vi "StartSweepMeasurement.vi"(8 "error in (no error)":errorcluster, 11 "9770 API in":refnum<class "9770 API.lvclass">) -> (0 "error out":errorcluster, 3 "9770 API out":refnum<class "9770 API.lvclass">)   [LabVIEW 2017, in "9770 API.lvclass"]
uses:
  <vilib>/addons/InsightCM/Devices/Shared/Emsa/Emsa9770API/9770 API.lvclass
  <vilib>/addons/InsightCM/Devices/Shared/Emsa/Emsa9770API/9770 API.lvclass/9770 API.ctl
  <vilib>/LabVIEW Targets/FPGA/cRIO/shared/nicrio_ModuleControls/nicrio_cRIO-9770_DataRatesRing.ctl
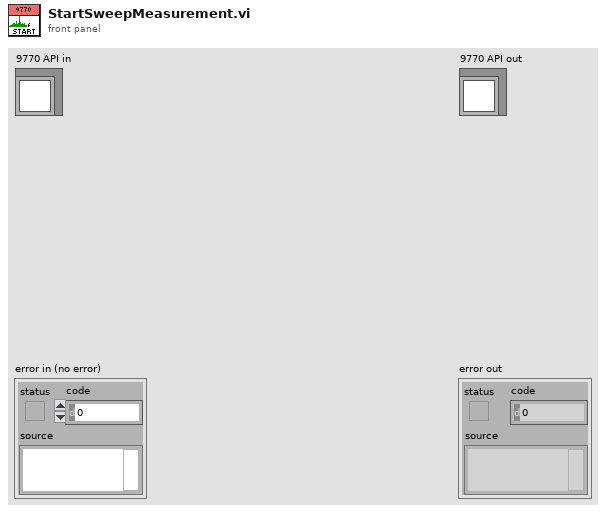
[diagram p1: front panel]
types:
  T1 = cluster{"Sweep":cluster{"Center Freq":dbl, "Bandwidth":dbl}[], "SampleRate":dbl, "FullScaleVoltage":dbl, "DetectionTime":dbl, "DetectionMode":enum16{"Peak", "Quasi Peak", "Average"}}
  T2 = typedef "nicrio_cRIO-9770_DataRatesRing.ctl" = u8
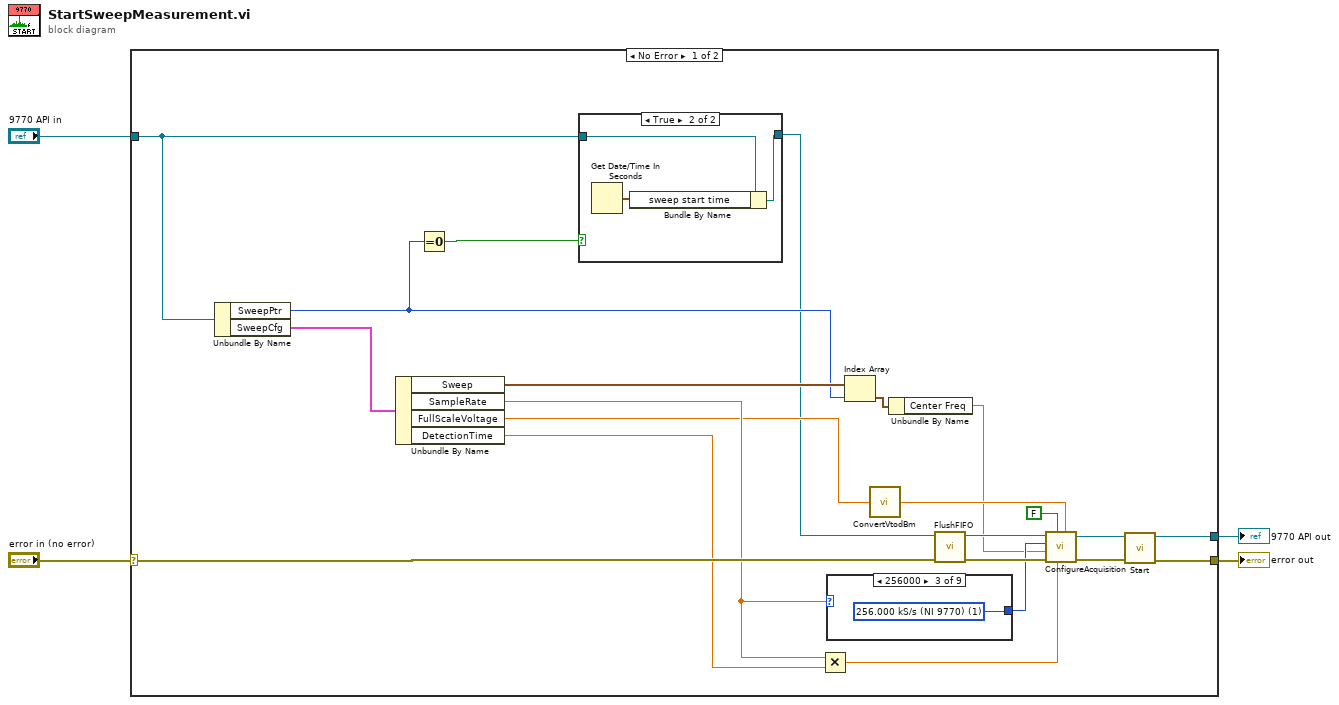
[diagram p0: block diagram]
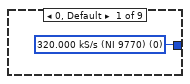
[diagram p3: hidden frame]
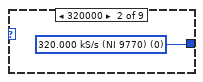
[diagram p4: hidden frame]
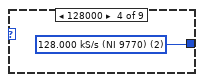
[diagram p5: hidden frame]
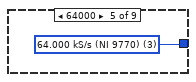
[diagram p6: hidden frame]
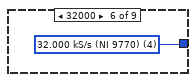
[diagram p7: hidden frame]
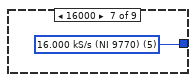
[diagram p8: hidden frame]
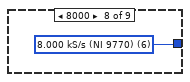
[diagram p9: hidden frame]
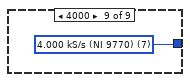
[diagram p10: hidden frame]
diagram:
  n1 = case shown="No Error" "error in (no error)" {
    selector: "error in (no error)" -> [w26 w41]
    tunnel: [w6 w41] -> w3
    tunnel: [w5 w40] -> w1
    tunnel: "9770 API in" -> [w9 w40]
    frame No Error {
      n2 = Unbundle By Name(w9) -> ("SweepPtr"=w11:i32, "SweepCfg"=w23:T1)
      n3 = Unbundle By Name(w23) -> ("Sweep"=w21:cluster{"Center Freq":dbl, "Bandwidth":dbl}[], "SampleRate"=w16:dbl, "FullScaleVoltage"=w13:dbl, "DetectionTime"=w19:dbl)
      n4 = Equal To 0?(x=w11) -> (x = 0?=w10:bool)
      n5 = case shown="True" w10 {
        tunnel: w9 -> [w27 w30]
        tunnel: [w27 w29] -> w8
        frame False {
        }
        frame True {
          n6 = Get Date/Time In Seconds() -> (seconds since 1Jan1904=w28:timestamp)
          n7 = Bundle By Name(cluster=w30, "sweep start time"=w28) -> (w29:refnum<class "9770 API.lvclass">)
        }
      }
      n8 = Multiply(x=w16, y=w19) -> (x*y=w18:dbl)
      n9 = case shown="256000" w16 {
        tunnel: [w31 w32 w33 w34 w35 w36 w37 w38 w39] -> w17
        frame 0, Default {
          w31 = T2 0 items=["320.000 kS/s (NI 9770)", "256.000 kS/s (NI 9770)", "128.000 kS/s (NI 9770)", "64.000 kS/s (NI 9770)", "32.000 kS/s (NI 9770)", "16.000 kS/s (NI 9770)", "8.000 kS/s (NI 9770)", "4.000 kS/s (NI 9770)"] ("Data Rate")
        }
        frame 320000 {
          w32 = T2 0 items=["320.000 kS/s (NI 9770)", "256.000 kS/s (NI 9770)", "128.000 kS/s (NI 9770)", "64.000 kS/s (NI 9770)", "32.000 kS/s (NI 9770)", "16.000 kS/s (NI 9770)", "8.000 kS/s (NI 9770)", "4.000 kS/s (NI 9770)"] ("Data Rate")
        }
        frame 256000 {
          w33 = T2 1 items=["320.000 kS/s (NI 9770)", "256.000 kS/s (NI 9770)", "128.000 kS/s (NI 9770)", "64.000 kS/s (NI 9770)", "32.000 kS/s (NI 9770)", "16.000 kS/s (NI 9770)", "8.000 kS/s (NI 9770)", "4.000 kS/s (NI 9770)"] ("Data Rate")
        }
        frame 128000 {
          w34 = T2 2 items=["320.000 kS/s (NI 9770)", "256.000 kS/s (NI 9770)", "128.000 kS/s (NI 9770)", "64.000 kS/s (NI 9770)", "32.000 kS/s (NI 9770)", "16.000 kS/s (NI 9770)", "8.000 kS/s (NI 9770)", "4.000 kS/s (NI 9770)"] ("Data Rate")
        }
        frame 64000 {
          w35 = T2 3 items=["320.000 kS/s (NI 9770)", "256.000 kS/s (NI 9770)", "128.000 kS/s (NI 9770)", "64.000 kS/s (NI 9770)", "32.000 kS/s (NI 9770)", "16.000 kS/s (NI 9770)", "8.000 kS/s (NI 9770)", "4.000 kS/s (NI 9770)"] ("Data Rate")
        }
        frame 32000 {
          w36 = T2 4 items=["320.000 kS/s (NI 9770)", "256.000 kS/s (NI 9770)", "128.000 kS/s (NI 9770)", "64.000 kS/s (NI 9770)", "32.000 kS/s (NI 9770)", "16.000 kS/s (NI 9770)", "8.000 kS/s (NI 9770)", "4.000 kS/s (NI 9770)"] ("Data Rate")
        }
        frame 16000 {
          w37 = T2 5 items=["320.000 kS/s (NI 9770)", "256.000 kS/s (NI 9770)", "128.000 kS/s (NI 9770)", "64.000 kS/s (NI 9770)", "32.000 kS/s (NI 9770)", "16.000 kS/s (NI 9770)", "8.000 kS/s (NI 9770)", "4.000 kS/s (NI 9770)"] ("Data Rate")
        }
        frame 8000 {
          w38 = T2 6 items=["320.000 kS/s (NI 9770)", "256.000 kS/s (NI 9770)", "128.000 kS/s (NI 9770)", "64.000 kS/s (NI 9770)", "32.000 kS/s (NI 9770)", "16.000 kS/s (NI 9770)", "8.000 kS/s (NI 9770)", "4.000 kS/s (NI 9770)"] ("Data Rate")
        }
        frame 4000 {
          w39 = T2 7 items=["320.000 kS/s (NI 9770)", "256.000 kS/s (NI 9770)", "128.000 kS/s (NI 9770)", "64.000 kS/s (NI 9770)", "32.000 kS/s (NI 9770)", "16.000 kS/s (NI 9770)", "8.000 kS/s (NI 9770)", "4.000 kS/s (NI 9770)"] ("Data Rate")
        }
      }
      n10 = Index Array(array=w21, index=w11) -> (element=w20:cluster{"Center Freq":dbl, "Bandwidth":dbl})
      n11 = call <vilib>:"ConvertVtodBm.vi"("voltage"=w13) -> ("dBm"=w12:dbl)  [unwired: 4 in]
      n12 = Unbundle By Name(w20) -> ("Center Freq"=w7:dbl)
      n13 = call <vilib>:"FlushFIFO.vi"("error in (no error)"=w26, "9770 API in"=w8) -> ("error out"=w25:errorcluster, "9770 API out"=w24:refnum<class "9770 API.lvclass">)  [unwired: 8 in]
      n14 = call <vilib>:"ConfigureAcquisition.vi"("Reference Level (dBm)"=w12, "Number of Samples"=w18, "Continuous"=FALSE, "error in (no error)"=w25, "Center Frequency (Hz)"=w7, "Data Rate"=w17, "9770 API in"=w24) -> ("error out"=w15:errorcluster, "9770 API out"=w14:refnum<class "9770 API.lvclass">)  [unwired: 3 in]
      n15 = call-dynamic "Start.vi"("error in (no error)"=w15, "RIO_API in"=w14) -> ("error out"=w6:errorcluster, "RIO_API out"=w5:refnum<class "9770 API.lvclass">)  [unwired: 8 in]
    }
    frame Error {
    }
  }
  "error out" <- w3
  "9770 API out" <- w1
